vi "Test.vi"() -> ()   [LabVIEW 2017]
uses:
  Example Actor.lvclass
  C:/Program Files (x86)/National Instruments/LabVIEW 2017/vi.lib/ActorFramework/Actor/Actor.lvclass
  <vilib>/NI/Event Source Actor/Event Source/Event/Event.lvclass/Event.ctl
  <vilib>/NI/Event Source Actor/Event Source/Event Source Messages/Generate Event Msg/Generate Event Msg.lvclass/Generate Event Msg.ctl
  <vilib>/ActorFramework/Message Enqueuer/Message Enqueuer.lvclass/Message Enqueuer.ctl
  09906144-883f-4ab8-a24e-6e768e552b17.vi
  <vilib>/ActorFramework/Message Enqueuer/Enqueue.vi
  <vilib>/NI/Event Source Actor/Event Source/Event Source Messages/Generate Event Msg/Generate Event Msg.lvclass
  C:/Program Files (x86)/National Instruments/LabVIEW 2017/vi.lib/ActorFramework/Message/Message.lvclass
  <vilib>/ActorFramework/Stop Msg/Stop Msg.lvclass
  <vilib>/Utility/LVClass/Get LV Class Name.vi
  <resource>/AFDebug/Generate Trace for Message.vi
  <vilib>/ActorFramework/Message Priority Queue/Priority Enqueue.vi
  <vilib>/NI/Event Source Actor/Event Source/Event/Event.lvclass
  GlobalStopActor/GlobalStopActor.lvclass
  <vilib>/ActorFramework/Actor/Actor.lvclass
panel:
  out "Error Out":errorcluster
  in  "stop":bool
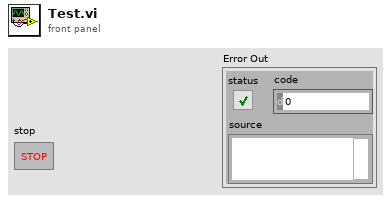
[diagram p1: front panel]
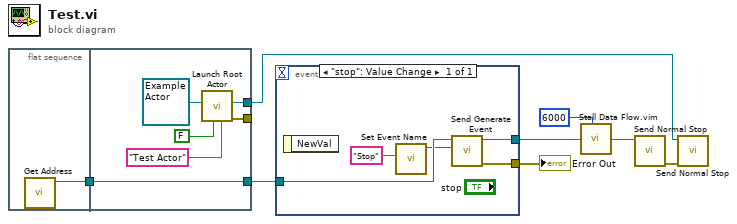
[diagram p0: block diagram]
diagram:
  n1 = flat-sequence {
    tunnel: [w9] -> w6
    tunnel: [w14] -> _
    tunnel: [w12] -> w5
    tunnel: w6 -> [w12]
    tunnel: [w10] -> w1
    frame #0 {
      n2 = call "Get Address.vi"() -> ("Enqueuer"=w9:refnum<class "Message Enqueuer.lvclass">)  [unwired: 11 in]
    }
    frame #1 {
      n3 = call <vilib>:"Launch Root Actor.vi"("Debug Alias"="Test Actor", "Open Actor Core front panel? (F)"=FALSE, "Actor"=refnum<class "Example Actor.lvclass"> refnum ("Example Actor.lvclass")) -> ("error out"=w14:errorcluster, "Actor's Enqueuer"=w10:refnum<class "Message Enqueuer.lvclass">)  [unwired: 7 in]
    }
  }
  n4 = event shown="[0] \"stop\": Value Change" {
    selector: _ -> [_]
    dyn-events: _ -> [_]
    timeout: _ -> [_]
    tunnel: [w17] -> w8
    tunnel: [w16] -> w7
    tunnel: w5 -> [w20]
    event "stop": Value Change {
      n5 = event-data() -> ()  [unwired: 1 in, 1 out]
      n6 = call <vilib>:"Set Event Name.vi"("Name (Generic)"="Stop") -> ("Event Out"=w19:refnum<class "Event.lvclass">)  [unwired: 10 in]
      n7 = call <vilib>:"Send Generate Event.vi"("Event"=w19, "Event Source Address"=w20) -> ("Error Out"=w16:errorcluster, "Event Source Address Out"=w17:refnum<class "Message Enqueuer.lvclass">)  [unwired: 8 in]
    }
  }
  "Error Out" <- w7
  n8 = call "Stall Data Flow.vim"("value in"=w8, "milliseconds to wait"=u32 6000) -> ("value out"=w4:refnum<class "Message Enqueuer.lvclass">)  [unwired: 1 out]
  n9 = call <vilib>:"Send Normal Stop.vi"("Message Enqueuer"=w4) -> ("error out"=w2:errorcluster)  [unwired: 10 in]
  n10 = call <vilib>:"Send Normal Stop.vi"("error in (no error)"=w2, "Message Enqueuer"=w1) -> ()  [unwired: 9 in, 1 out]
